vi "Autotest.vi"(8 "error in (no error)":errorcluster caption="entrée d'erreur (pas d'erreur)", 11 "Class Shielding_ Box JC-PB3044 en entrée":refnum<class "Class Shielding_ Box JC-PB3044.lvclass">) -> (0 "error out":errorcluster caption="sortie d'erreur", 2 "Autotest Ok":bool, 3 "Class Shielding_ Box JC-PB3044 en sortie":refnum<class "Class Shielding_ Box JC-PB3044.lvclass">)   [LabVIEW 2020, in "Library Instrument & Equipement.lvlib" / "Library Shielding box.lvlib" / "Class Shielding_ Box JC-PB3044.lvclass"]
uses:
  Class Shielding_ Box JC-PB3044.lvclass
  C:/Users/ngarcin/OneDrive - Altyor/Standard TB/Class/Shielding box/Class Shielding box (Default)/Class Shielding_ Box (Default).lvclass
  <vilib>/Instr/_visa.llb/VISA Find Search Mode.ctl
  Class Shielding_ Box JC-PB3044.lvclass/Class Shielding_ Box JC-PB3044.ctl
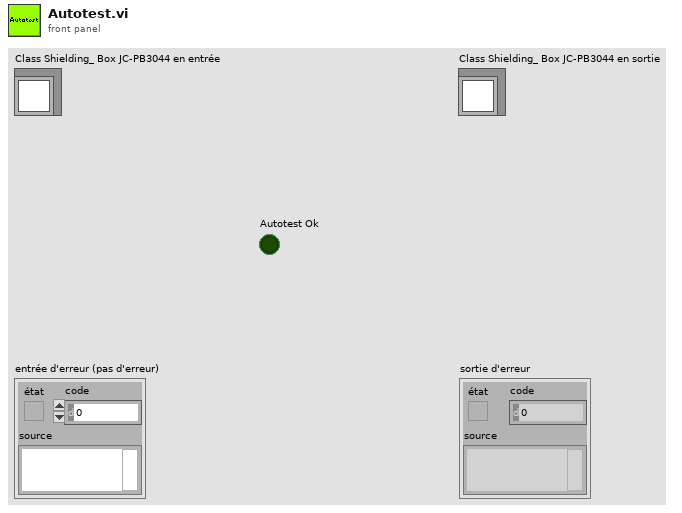
[diagram p1: front panel]
types:
  T1 = typedef "VISA Find Search Mode.ctl" = u32
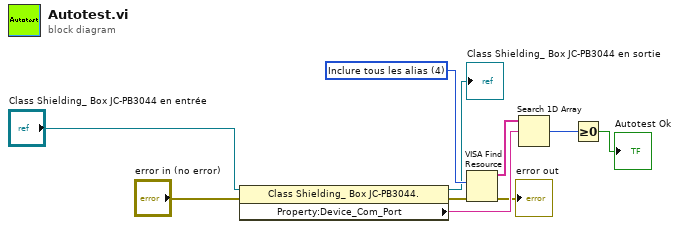
[diagram p0: block diagram]
diagram:
  w9 = T1 4 items=["Noms canoniques uniquement"=0, "Alias uniquement"=2, "Inclure les alias correspondants"=3, "Inclure tous les alias"=4] ("Search Mode")
  n1 = property class="Class Shielding_ Box JC-PB3044."(reference="Class Shielding_ Box JC-PB3044 en entrée", error in="error in (no error)") -> (reference out=→"Class Shielding_ Box JC-PB3044 en sortie":refnum<class "Class Shielding_ Box JC-PB3044.lvclass">, error out=w10:errorcluster, "Property:Device_Com_Port"=w8:string)
  n2 = VISA Find Resource(8:w10, 10:w9) -> (0:→"error out":errorcluster, 3:w7:string[])  [unwired: 1 in, 1 out]
  n3 = Search 1D Array(1D array=w7, element=w8) -> (index of element=w6:i32)  [unwired: 1 in]
  n4 = Greater Or Equal To 0?(x=w6) -> (x >= 0?=→"Autotest Ok":bool)
